vi "5668 Configure RF with External LO.vi"(8 "error in":errorcluster, 11 "Config Data in":T1={"Resource Name RFSA"="PXI1Slot13", "Resource Name RFSG LO Generation"="PXI1Slot9", " Start Carrier Frequency (Hz)"=4000000000.0, "Stop Carrier Frequency (Hz)"=6000000000.0, "Reference Level (dBm)"=0.0, "Resolution Bandwidth (Hz)"=10000.0} {"Resolution Bandwidth (Hz)" format="%#_6p"; "Reference Level (dBm)" format="%.2f"; "Stop Carrier Frequency (Hz)" format="%#_6p"; "Start Carrier Frequency (Hz)" format="%#_6p"}) -> (0 "error out":errorcluster, 3 "Config Data Out":T1={"Resource Name RFSA"="RFSA", "Resource Name RFSG LO Generation"="RFSG", " Start Carrier Frequency (Hz)"=4000000000.0, "Stop Carrier Frequency (Hz)"=6000000000.0, "Reference Level (dBm)"=0.0, "Resolution Bandwidth (Hz)"=10000.0} {"Resolution Bandwidth (Hz)" format="%#_6p"; "Reference Level (dBm)" format="%.2f"; "Stop Carrier Frequency (Hz)" format="%#_6p"; "Start Carrier Frequency (Hz)" format="%#_6p"})   [LabVIEW 2017]
uses:
  Config Data.ctl
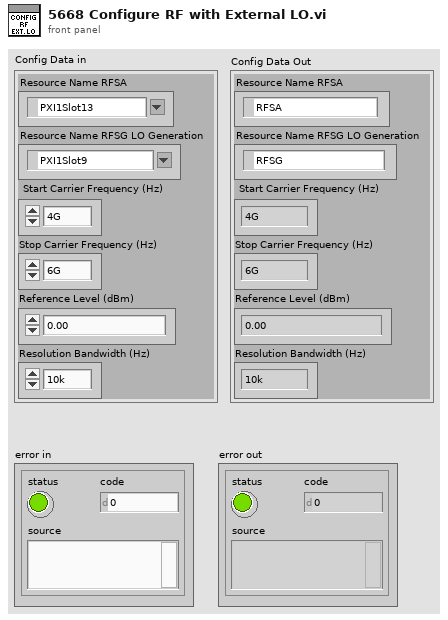
[diagram p1: front panel]
types:
  T1 = typedef "Config Data.ctl" = cluster{"Resource Name RFSA":refnum<k15>, "Resource Name RFSG LO Generation":refnum<k15>, " Start Carrier Frequency (Hz)":dbl, "Stop Carrier Frequency (Hz)":dbl, "Reference Level (dBm)":dbl, "Resolution Bandwidth (Hz)":dbl}
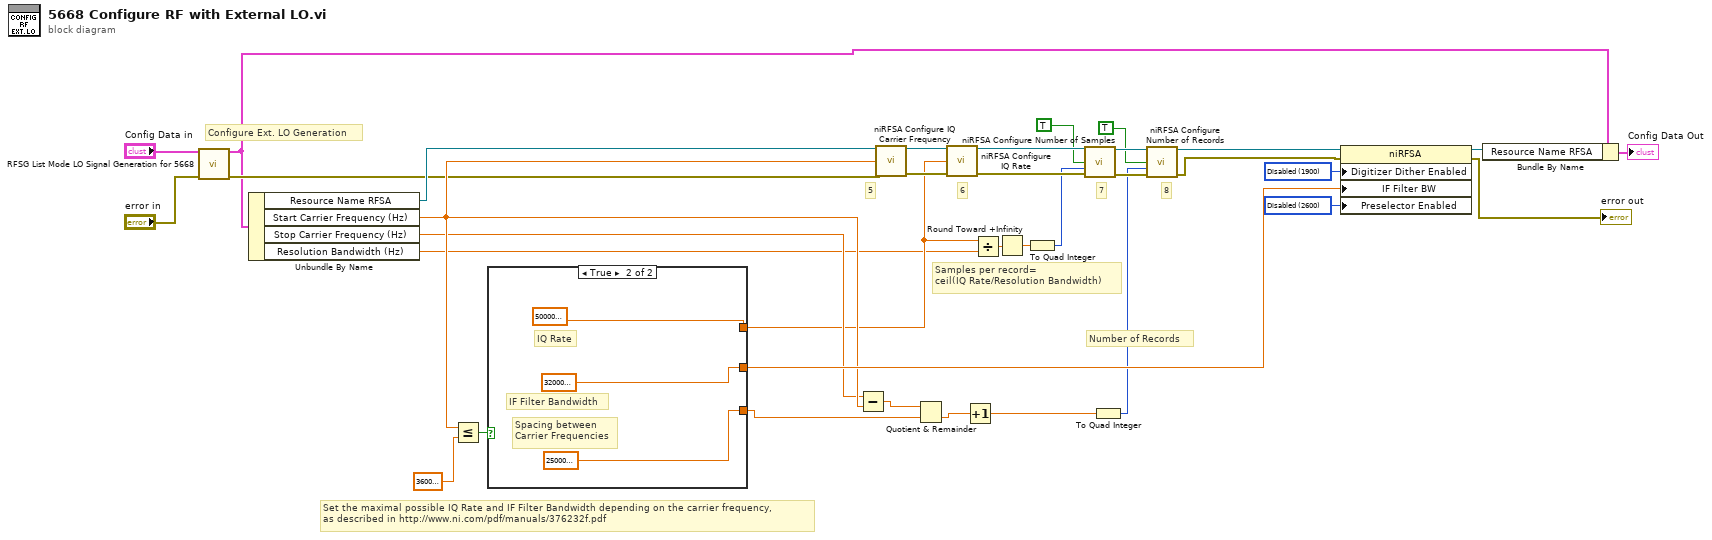
[diagram p0: block diagram]
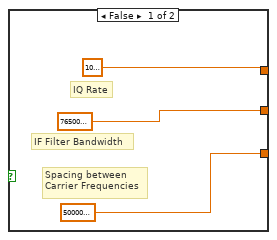
[diagram p2: hidden frame]
diagram:
  w23 = 2600 items=["Disabled"=2600, "Enabled when in Signal Path"=2601, "Enabled"=2602] ("Signal Path:Advanced:Downconverter Preselector Enabled")
  w24 = 1900 items=["Disabled"=1900, "Enabled"=1901] ("Signal Path:Digitizer Dither Enabled")
  # "Configure Ext. LO Generation"
  # "Number of Records"
  # "Samples per record= \nceil(IQ Rate/Resolution Bandwidth)"
  # "Set the maximal possible IQ Rate and IF Filter Bandwidth depending on the carrier frequency, \nas described in http://www.ni.com/pdf/manuals/376232f.pdf"
  # "8"
  # "7"
  # "6"
  # "5"
  n1 = call "RFSG List Mode LO Signal Generation for 5668.vi"("Config Data in"="Config Data in", "error in"="error in") -> ("Config Data Out"=w3:T1, "error out"=w5:errorcluster)  [unwired: 12 in]
  n2 = Unbundle By Name(w3) -> ("Resource Name RFSA"=w25:refnum<k15>, "Start Carrier Frequency (Hz)"=w17:dbl, "Stop Carrier Frequency (Hz)"=w16:dbl, "Resolution Bandwidth (Hz)"=w10:dbl)
  n3 = Less Or Equal?(x=w17, y=3600000000.0) -> (x <= y?=w11:bool)
  n4 = case shown="True" w11 {
    tunnel: [765000000.0 ("Signal Path:IF Filter Bandwidth") 320000000.0 ("Signal Path:IF Filter Bandwidth")] -> w22
    tunnel: [1000000000.0 ("IQ rate (S/s)") 500000000.0 ("IQ rate (S/s)")] -> w12
    tunnel: [500000000.0 ("Signal Path:IF Filter Bandwidth") 250000000.0 ("Signal Path:IF Filter Bandwidth")] -> w8
    frame False {
      # "Spacing between\nCarrier Frequencies"
      # "IF Filter Bandwidth"
      # "IQ Rate"
    }
    frame True {
      # "Spacing between\nCarrier Frequencies"
      # "IF Filter Bandwidth"
      # "IQ Rate"
    }
  }
  n5 = Subtract(x=w16, y=w17) -> (x-y=w20:dbl)
  n6 = call <instrlib>:"niRFSA Configure IQ Carrier Frequency.vi"("instrument handle"=w25, "carrier frequency"=w17, "error in"=w5) -> ("instrument handle out"=w29:refnum<k15>, "error out"=w28:errorcluster)  [unwired: 11 in]
  n7 = Quotient & Remainder(x=w20, y=w8) -> (floor(x/y)=w18:dbl)  [unwired: 1 out]
  n8 = call <instrlib>:"niRFSA Configure IQ Rate.vi"("instrument handle"=w29, "IQ rate (S/s)"=w12, "error in"=w28) -> ("instrument handle out"=w34:refnum<k15>, "error out"=w35:errorcluster)  [unwired: 11 in]
  n9 = Increment(x=w18) -> (x+1=w19:dbl)
  n10 = Divide(x=w12, y=w10) -> (x/y=w13:dbl)
  n11 = Round Toward +Infinity(x=w13) -> (ceil(x): smallest int >= x=w14:dbl)
  n12 = To Quad Integer(1:w14) -> (0:w9:i64)
  n13 = call <instrlib>:"niRFSA Configure Number of Samples.vi"("instrument handle"=w34, "number of samples is finite"=TRUE, "samples per record"=w9, "error in"=w35) -> ("instrument handle out"=w32:refnum<k15>, "error out"=w31:errorcluster)  [unwired: 10 in]
  n14 = To Quad Integer(1:w19) -> (0:w15:i64)
  n15 = call <instrlib>:"niRFSA Configure Number of Records.vi"("instrument handle"=w32, "number of records is finite"=TRUE, "number of records"=w15, "error in"=w31) -> ("instrument handle out"=w27:refnum<k15>, "error out"=w21:errorcluster)  [unwired: 10 in]
  n16 = property class="niRFSA"(reference=w27, error in=w21, "Digitizer Dither Enabled"=w24, "IF Filter BW"=w22, "Preselector Enabled"=w23) -> (reference out=w4:refnum<k15>, error out=→"error out":errorcluster)
  n17 = Bundle By Name(cluster=w3, "Resource Name RFSA"=w4) -> (→"Config Data Out":T1)
